vi "Fast Log VI v0.1.vi"() -> ()   [LabVIEW 2017]
uses:
  <vilib>/DAQmx/configure/timing.llb/DAQmx Timing (Use Waveform).vi
  <vilib>/DAQmx/create/channels.llb/DAQmx Create Channel (AO-Voltage-Basic).vi
  <vilib>/measure/NI_MABase.lvlib
  <vilib>/DAQmx/write.llb/DAQmx Write (Analog Wfm 1Chan NSamp).vi
  <resource>/objmgr/daqmx.rc
panel:
  out "Waveform Chart":dbl(graph)
  out "array":dbl[](array[numeric])
  out "Waveform Graph":waveform(dbl)(graph)
  in  "sample mode":i32(ring)=10178 items=["Finite Samples"=10178, "Continuous Samples"=10123, "Hardware Timed Single Point"=12522]
  out "number of samples written per channel":u32
  in  "sampling info":cluster{"Fs":dbl, "#s":dbl}={"Fs"=1000.0, "#s"=1000.0} {"Fs" format="%.2p"}
  in  "maximum value":dbl=10.0 format="%0.2f"
  in  "minimum value":dbl=-10.0 format="%0.2f"
  in  "frequency":dbl=10.0 format="%0.2p"
  in  "amplitude":dbl=1.0 format="%0.2p"
  in  "phase":dbl format="%.2p"
  in  "offset":dbl format="%0.2p V"
  in  "Physical Channels 2":tag="Dev1/ao1"
  in  "error in (no error)":errorcluster
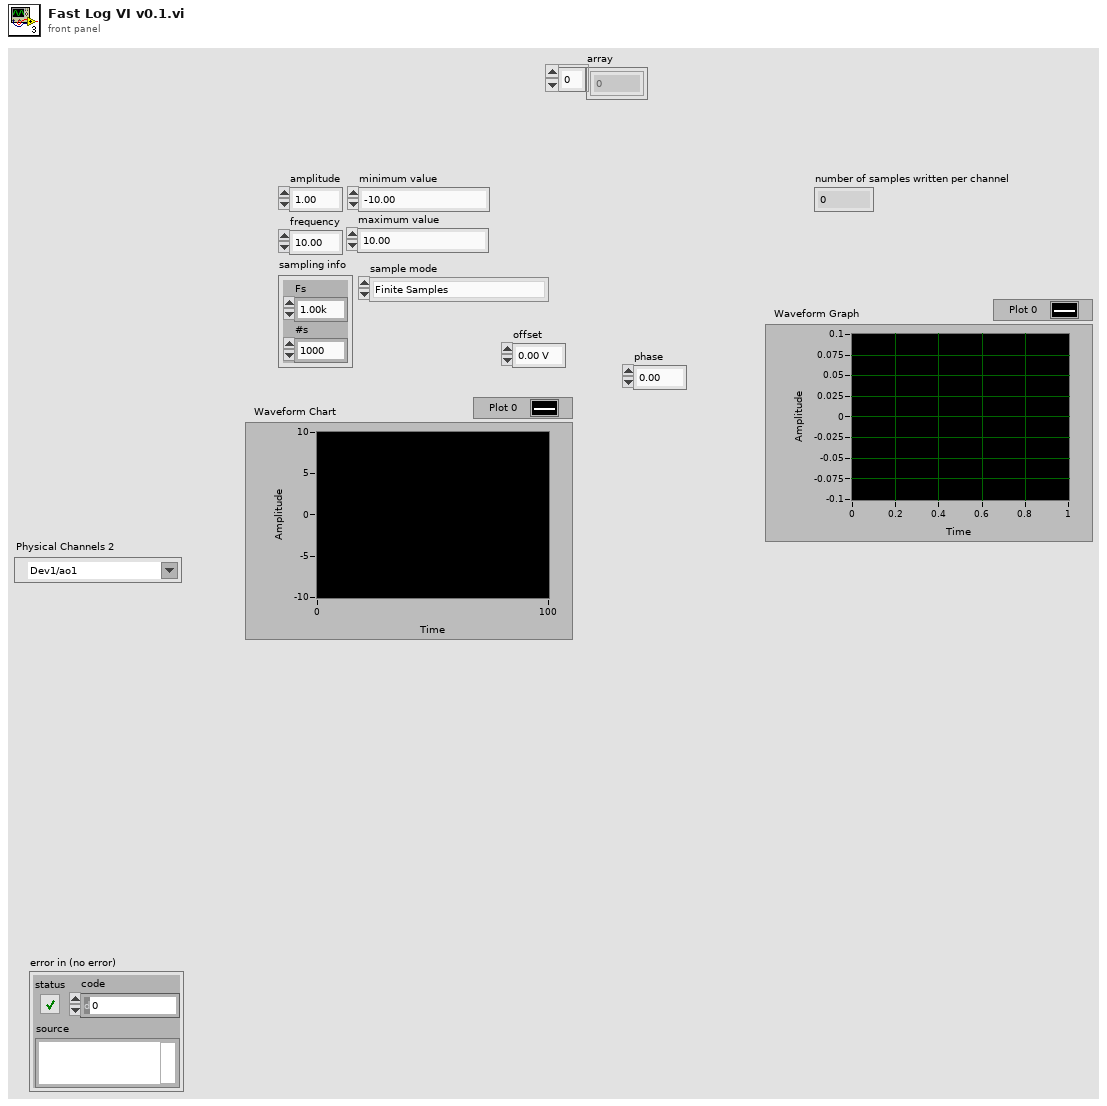
[diagram p1: front panel]
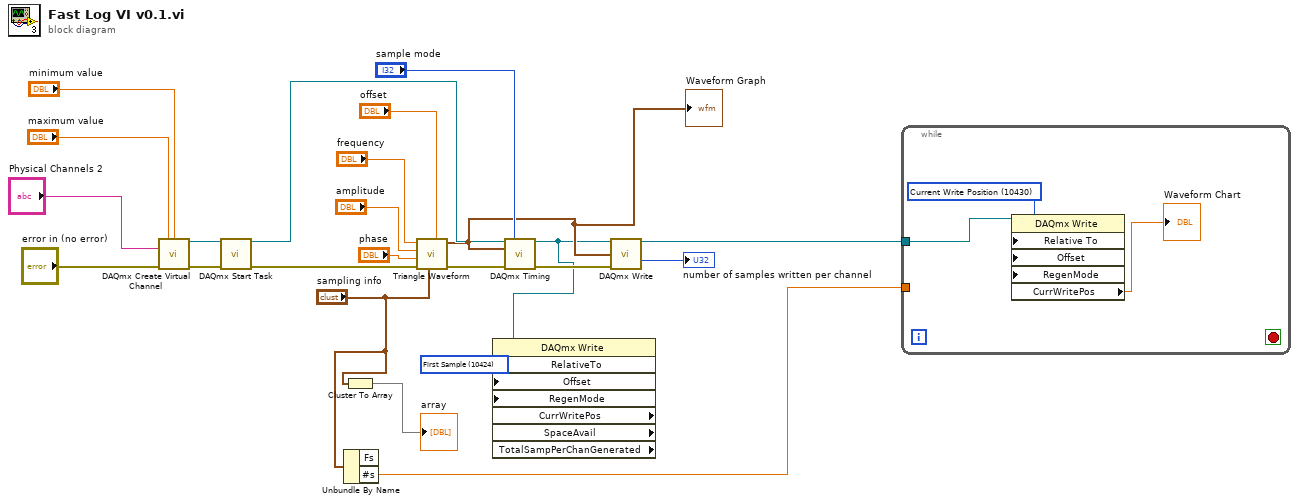
[diagram p0: block diagram]
diagram:
  w1 = 10424 items=["First Sample"=10424, "Current Write Position"=10430] ("RelativeTo")
  n1 = call-poly <vilib>:"DAQmx Create Virtual Channel.vi"("maximum value"="maximum value", "minimum value"="minimum value", "physical channels"="Physical Channels 2", "error in"="error in (no error)") -> ("task out"=w21:refnum<k21>, "error out"=w20:errorcluster)  [unwired: 10 in]
  n2 = call <vilib>:"DAQmx Start Task.vi"("task/channels in"=w21, "error in"=w20) -> ("task out"=w18:refnum<k21>, "error out"=w19:errorcluster)  [unwired: 12 in]
  n3 = Unbundle By Name("sampling info") -> ("#s"=w3:dbl)  [unwired: 1 out]
  n4 = Cluster To Array(cluster="sampling info") -> (array=→"array":dbl[])
  n5 = call <vilib>:"Triangle Waveform.vi"("offset"="offset", "sampling info"="sampling info", "error in (no error)"=w19, "phase"="phase", "amplitude"="amplitude", "frequency"="frequency") -> ("error out"=w11:errorcluster, "signal out"=w7:waveform(dbl))  [unwired: 4 in]
  "Waveform Graph" <- w7
  n6 = call-poly <vilib>:"DAQmx Timing.vi"("task/channels in"=w18, "sample mode"="sample mode", "waveform"=w7, "error in"=w11) -> ("task out"=w2:refnum<k21>, "error out"=w10:errorcluster)  [unwired: 10 in]
  n7 = property class="DAQmx Write" props=["RelativeTo", "Offset", "RegenMode", "CurrWritePos", "SpaceAvail", "TotalSampPerChanGenerated"](reference=w2, "RelativeTo"=w1) -> ()  [unwired: 3 in, 5 out]
  n8 = call-poly <vilib>:"DAQmx Write.vi"("task/channels in"=w2, "data"=w7, "error in"=w10) -> ("task out"=w6:refnum<k21>, "number of samples written per channel"=→"number of samples written per channel":u32)  [unwired: 10 in, 1 out]
  n9 = while {
    tunnel: w6 -> [w25]
    tunnel: w3 -> [_]
    stop <- _ stop-if-true
    w26 = 10430 items=["First Sample"=10424, "Current Write Position"=10430] ("RelativeTo")
    n10 = property class="DAQmx Write" props=["Relative To", "Offset", "RegenMode", "CurrWritePos"](reference=w25, "Relative To"=w26) -> ("CurrWritePos"=→"Waveform Chart":dbl)  [unwired: 3 in, 2 out]
  }
